vi "Set Default Configuration.vi"(8 "error in":errorcluster, 11 "EMS Generic in":refnum<class "EMS Generic.lvclass">) -> (0 "error out":errorcluster, 3 "EMS Generic out":refnum<class "EMS Generic.lvclass">)   [LabVIEW 2018, in "EMS Generic Actor.lvlib" / "EMS Generic.lvclass"]
uses:
  EMS Generic.lvclass
  EMS Generic.lvclass/EMS Generic.ctl
  <vilib>/Utility/config.llb/Write Key (Path).vi
  <vilib>/Utility/config.llb/NI_LVConfig.lvlib
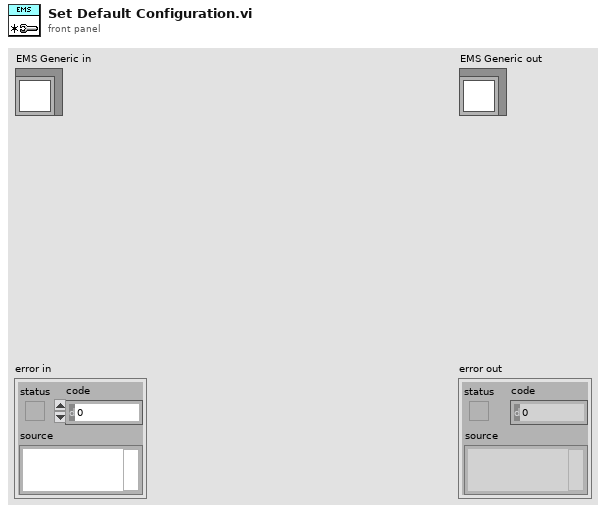
[diagram p1: front panel]
types:
  T1 = typedef "NI_LVConfig.lvlib/Config Data RefNum.ctl" = refnum<k1>
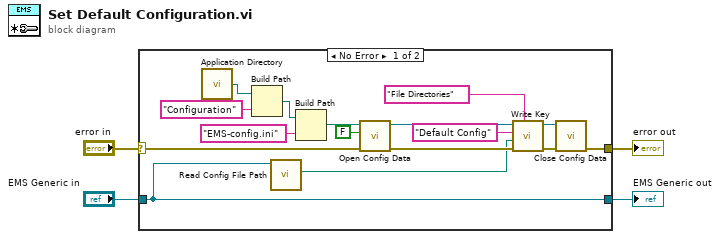
[diagram p0: block diagram]
diagram:
  n1 = case shown="No Error" "error in" {
    selector: "error in" -> [w14 w22]
    tunnel: [w7 w22] -> w3
    tunnel: [w6 w21] -> w1
    tunnel: "EMS Generic in" -> [w6 w21]
    frame No Error {
      n2 = call <vilib>:"Application Directory.vi"() -> ("Application Directory"=w16:path)
      n3 = Build Path(base path=w16, name or relative path="Configuration") -> (appended path=w17:path)
      n4 = call "Read Config File Path.vi"("EMS Generic in"=w6) -> ("Config File Path"=w5:path)  [unwired: 8 in, 2 out]
      n5 = Build Path(base path=w17, name or relative path="EMS-config.ini") -> (appended path=w19:path)
      n6 = call <vilib>:"Open Config Data.vi"("error in (no error)"=w14, "create file if necessary (T)"=FALSE, "configuration file path"=w19) -> ("error out"=w10:errorcluster, "refnum"=w11:T1)  [unwired: 6 in, 1 out]
      n7 = call-poly <vilib>:"Write Key.vi"("section"="File Directories", "error in (no error)"=w10, "value"=w5, "key"="Default Config", "refnum"=w11) -> ("error out"=w8:errorcluster, "refnum out"=w9:T1)  [unwired: 4 in, 1 out]
      n8 = call <vilib>:"Close Config Data.vi"("error in (no error)"=w8, "refnum"=w9) -> ("error out"=w7:errorcluster)  [unwired: 8 in, 1 out]
    }
    frame Error {
    }
  }
  "error out" <- w3
  "EMS Generic out" <- w1
